vi "reward_behavior_0_6s_post_stim.vi"() -> ()   [LabVIEW 2019]
doc: "The myRIO Project template acquires acceleration data from the onboard accelerometer and displays the changes of acceleration values in a waveform chart."
uses:
  <vilib>/Analysis/Matrix/Datatypes/RealMatrix.ctl
  <vilib>/myRIO/Common/Instrument Driver Framework/myRIO v1.0/Encoder/typedefs/Encoder Signal Mode.ctl
  <vilib>/myRIO/Instrument Drivers/Onboard IO/Encoder/typedefs/Encoder Reference.ctl
  <vilib>/myRIO/Common/Instrument Driver Framework/Utilities/typedefs/myRIO Generic Hardware Reference.ctl
  <vilib>/myRIO/Common/Instrument Driver Framework/Utilities/typedefs/Hardware Version Enum.ctl
  <vilib>/myRIO/Common/Instrument Driver Framework/Utilities/typedefs/myRIO v1.0 Reference.ctl
  <vilib>/myRIO/Common/Instrument Driver Framework/Utilities/typedefs/Generic FPGA Reference.ctl
  <vilib>/myRIO/Common/Instrument Driver Framework/myRIO v1.0/Encoder/typedefs/Encoder Channels Enum.ctl
  <vilib>/myRIO/Common/Instrument Driver Framework/myRIO v1.0/Encoder/typedefs/Encoder Configuration v1.0.ctl
  <vilib>/userdefined/High Color/nirio_resource_hc.ctl
  <vilib>/myRIO/Instrument Drivers/Onboard IO/DIO/typedefs/DIO Reference.ctl
  <vilib>/myRIO/Common/Instrument Driver Framework/myRIO v1.0/DIO/typedefs/DIO Channels List.ctl
  <vilib>/myRIO/Common/Instrument Driver Framework/myRIO v1.0/DIO/typedefs/DIO Channels Enum.ctl
  <vilib>/myRIO/Common/Instrument Driver Framework/Utilities/vis/Is FPGA Ref Available.vi
  <vilib>/myRIO/Common/Instrument Driver Framework/myRIO v1.0/Encoder/vis/myRIO v1.1 Open Encoder.vi
  <vilib>/myRIO/Instrument Drivers/Onboard IO/Encoder/vis/Read.vi
  <vilib>/myRIO/Common/Instrument Driver Framework/myRIO v1.0/DIO/vis/myRIO v1.1 Open DIO.vi
  <vilib>/myRIO/Instrument Drivers/Onboard IO/DIO/vis/Write.vi
  <vilib>/myRIO/Instrument Drivers/Onboard IO/DIO/vis/Read.vi
  <vilib>/myRIO/Common/Instrument Driver Framework/Utilities/vis/Validate Channels.vi
  <vilib>/myRIO/Common/Instrument Driver Framework/myRIO v1.0/Encoder/vis/myRIO v1.0 Reserve Encoder.vi
  <vilib>/myRIO/Common/Instrument Driver Framework/myRIO v1.0/DIO/vis/myRIO v1.0 Reserve DIO.vi
  <vilib>/myRIO/Common/Instrument Driver Framework/myRIO v1.0/Encoder/vis/myRIO v1.0 Build MUX Configuration Encoder.vi
  <vilib>/myRIO/Common/Instrument Driver Framework/myRIO v1.0/Resource Manager/vis/myRIO v1.0 Reserve Channel List.vi
  <vilib>/myRIO/Common/Instrument Driver Framework/myRIO v1.0/DIO/vis/myRIO v1.0 Build MUX Configuration DIO.vi
  <vilib>/myRIO/Common/Instrument Driver Framework/myRIO v1.0/Resource Manager/vis/myRIO v1.0 Create Configuration List.vi
  <vilib>/myRIO/Common/Instrument Driver Framework/myRIO v1.0/Resource Manager/vis/myRIO v1.0 Reserve Channel.vi
  <vilib>/myRIO/Common/Instrument Driver Framework/myRIO v1.0/Resource Manager/vis/myRIO v1.0 Unreserve Channel.vi
  <vilib>/myRIO/Common/Instrument Driver Framework/myRIO v1.0/Resource Manager/vis/myRIO v1.0 Build Mutex Name.vi
  <vilib>/Utility/VariantDataType/GetNumericInfo.vi
  <vilib>/Utility/error.llb/Error Cluster From Error Code.vi
  <vilib>/myRIO/Common/Instrument Driver Framework/myRIO v1.0/myRIO v1.1 Open.vi
  <vilib>/myRIO/Common/Instrument Driver Framework/Utilities/vis/IO Manager.vi
  <vilib>/myRIO/Common/Instrument Driver Framework/Utilities/vis/Configuration Manager.vi
  <vilib>/myRIO/Common/Instrument Driver Framework/myRIO v1.0/Resource Manager/vis/myRIO v1.0 Configure IO.vi
  <vilib>/myRIO/Common/Instrument Driver Framework/myRIO v1.0/myRIO v1.0 Close.vi
  <vilib>/myRIO/Common/Instrument Driver Framework/myRIO v1.0/Encoder/vis/myRIO v1.0 Configure Encoder.vi
  <vilib>/myRIO/Common/Instrument Driver Framework/myRIO v1.0/Encoder/vis/myRIO v1.0 Read Encoder.vi
  <vilib>/myRIO/Common/Instrument Driver Framework/myRIO v1.0/DIO/vis/myRIO v1.0 Read DIO.vi
  <vilib>/myRIO/Common/Instrument Driver Framework/myRIO v1.0/DIO/vis/myRIO v1.0 Write DIO.vi
  <vilib>/myRIO/Express VI/Onboard IO/Encoder/Encoder Express VI.xnode
  <vilib>/myRIO/Instrument Drivers/Onboard IO/Encoder/vis/myRIO Encoder Open.xnode
  <vilib>/myRIO/Express VI/Onboard IO/DI/DI Express VI.xnode
  <vilib>/myRIO/Instrument Drivers/Onboard IO/DIO/vis/myRIO DIO Open.xnode
  <vilib>/myRIO/Express VI/Onboard IO/DO/DO Express VI.xnode
  <vilib>/myRIO/Instrument Drivers/Onboard IO/Encoder/Encoder.lvlib
  <vilib>/myRIO/Instrument Drivers/Onboard IO/DIO/DIO.lvlib
  <vilib>/Analysis/Matrix/NI_Matrix.lvlib
panel:
  out "Rewarded trials":dbl[](array[numeric])
  out "Rewards":u16
  out "Active Trial":bool
  out "Array temp2":T1
  out "Stimuli Loaded":bool
  out "Stim_ID":dbl[](array[numeric])
  out "Reward_mat":dbl[](array[numeric])
  out "Reward":bool=TRUE
  out "Frame clock":i32
  out "Licks":u32
  out "Lick":bool
  out "Time":dbl
  out "Stop":bool
  in  "Frames to collect":u32
  out "Overflow?":bool
  out "Counter Value":i32
  out "Velocity":dbl
  out "Velocity Plot":dbl[](graph)
  out "Velocity array":dbl[](array[numeric])
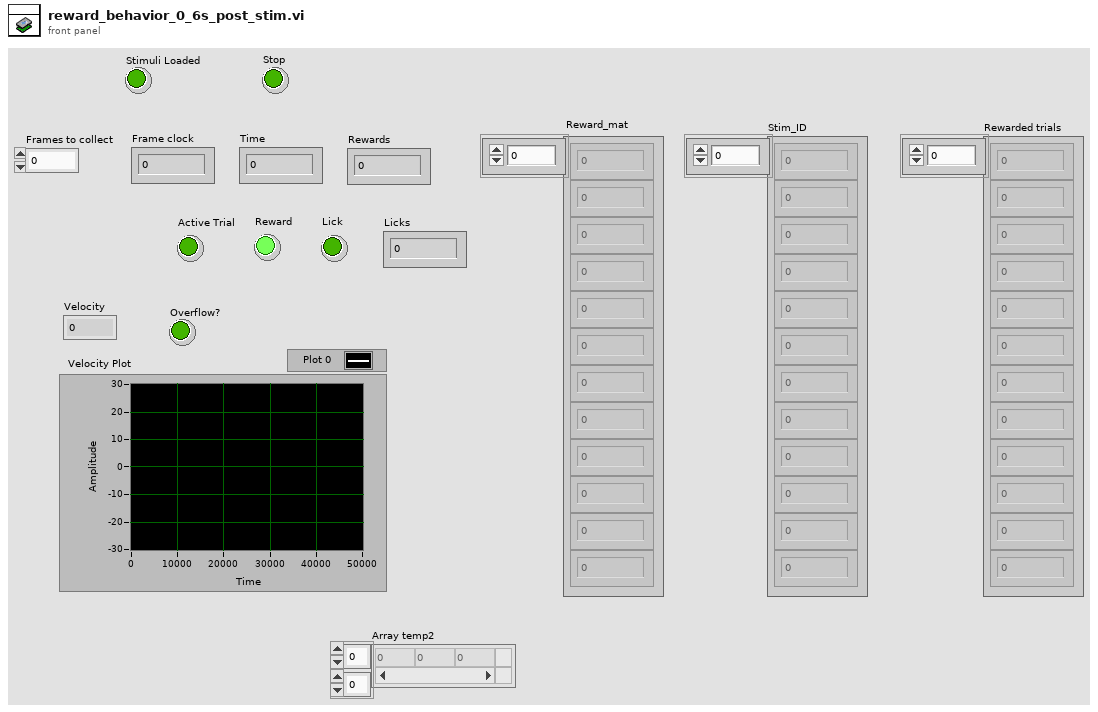
[diagram p1: front panel]
types:
  T1 = typedef "NI_Matrix.lvlib/RealMatrix.ctl" = dbl[][]
  T2 = typedef "Encoder.lvlib/Encoder Reference.ctl" = cluster{"myRIO Reference":T3, "Encoder Channels Enum":T7}
  T3 = typedef "myRIO Generic Hardware Reference.ctl" = cluster{"myRIO Model":T4, "myRIO Hardware Reference":T5}
  T4 = typedef "Hardware Version Enum.ctl" = enum16{"Unknown", "myRIO-1900", "myRIO-1950", "roboRIO", "NI ELVIS RIO CM", "ELVIS III"}
  T5 = typedef "myRIO v1.0 Reference.ctl" = cluster{"Generic FPGA Reference":T6, "Allow multiple opens":bool}
  T6 = typedef "Generic FPGA Reference.ctl" = refnum<k20>
  T7 = typedef "Encoder Channels Enum.ctl" = enum16{"Not Connected", "C/ENC0", "C/ENC1", "A/ENC", "A/ENC0", "A/ENC1", "A/ENC2", "A/ENC3", "A/ENC4", "A/ENC5", "A/ENC6", "A/ENC7", "A/ENC8", "A/ENC9", "B/ENC", "B/ENC0", "B/ENC1", "B/ENC2", "B/ENC3", "B/ENC4", "B/ENC5", "B/ENC6", "B/ENC7", "B/ENC8", "B/ENC9", "DIO/ENC0", "DIO/ENC1", "DIO/ENC2", "DIO/ENC3", "DIO/ENC4"}
  T8 = typedef "Encoder Signal Mode.ctl" = enum16{"Quadrature phase signal", "Step and direction signal"}
  T9 = typedef "nirio_resource_hc.ctl" = tag
  T10 = typedef "DIO.lvlib/DIO Reference.ctl" = cluster{"myRIO Reference":T3, "DIO Channels List":T11}
  T11 = typedef "DIO Channels List.ctl" = T12[]
  T12 = typedef "DIO Channels Enum.ctl" = enum16{"Not Connected", "C/DIO0", "C/DIO1", "C/DIO2", "C/DIO3", "C/DIO4", "C/DIO5", "C/DIO6", "C/DIO7", "A/DIO0", "A/DIO1", "A/DIO2", "A/DIO3", "A/DIO4", "A/DIO5", "A/DIO6", "A/DIO7", "A/DIO8", "A/DIO9", "A/DIO10", "A/DIO11", "A/DIO12", "A/DIO13", "A/DIO14", "A/DIO15", "A/DIO16", "A/DIO17", "A/DIO18", "A/DIO19", "B/DIO0", "B/DIO1", "B/DIO2", "B/DIO3", "B/DIO4", "B/DIO5", "B/DIO6", "B/DIO7", "B/DIO8", "B/DIO9", "B/DIO10", "B/DIO11", "B/DIO12", "B/DIO13", "B/DIO14", "B/DIO15", "B/DIO16", "B/DIO17", "B/DIO18", "B/DIO19", "LED0", "LED1", "LED2", "LED3", "Button0", "DIO/DIO0", "DIO/DIO1", "DIO/DIO2", "DIO/DIO3", "DIO/DIO4", "DIO/DIO5", "DIO/DIO6", "DIO/DIO7", "DIO/DIO8", "DIO/DIO9", "SPI/CS0", "SPI/CS1", "SPI/CS2", "SPI/CS3", "LED RADIO (Green)", "LED RADIO (Red)", "LED COMM (Green)", "LED COMM (Red)", "LED MODE (Green)", "LED MODE (Red)"}
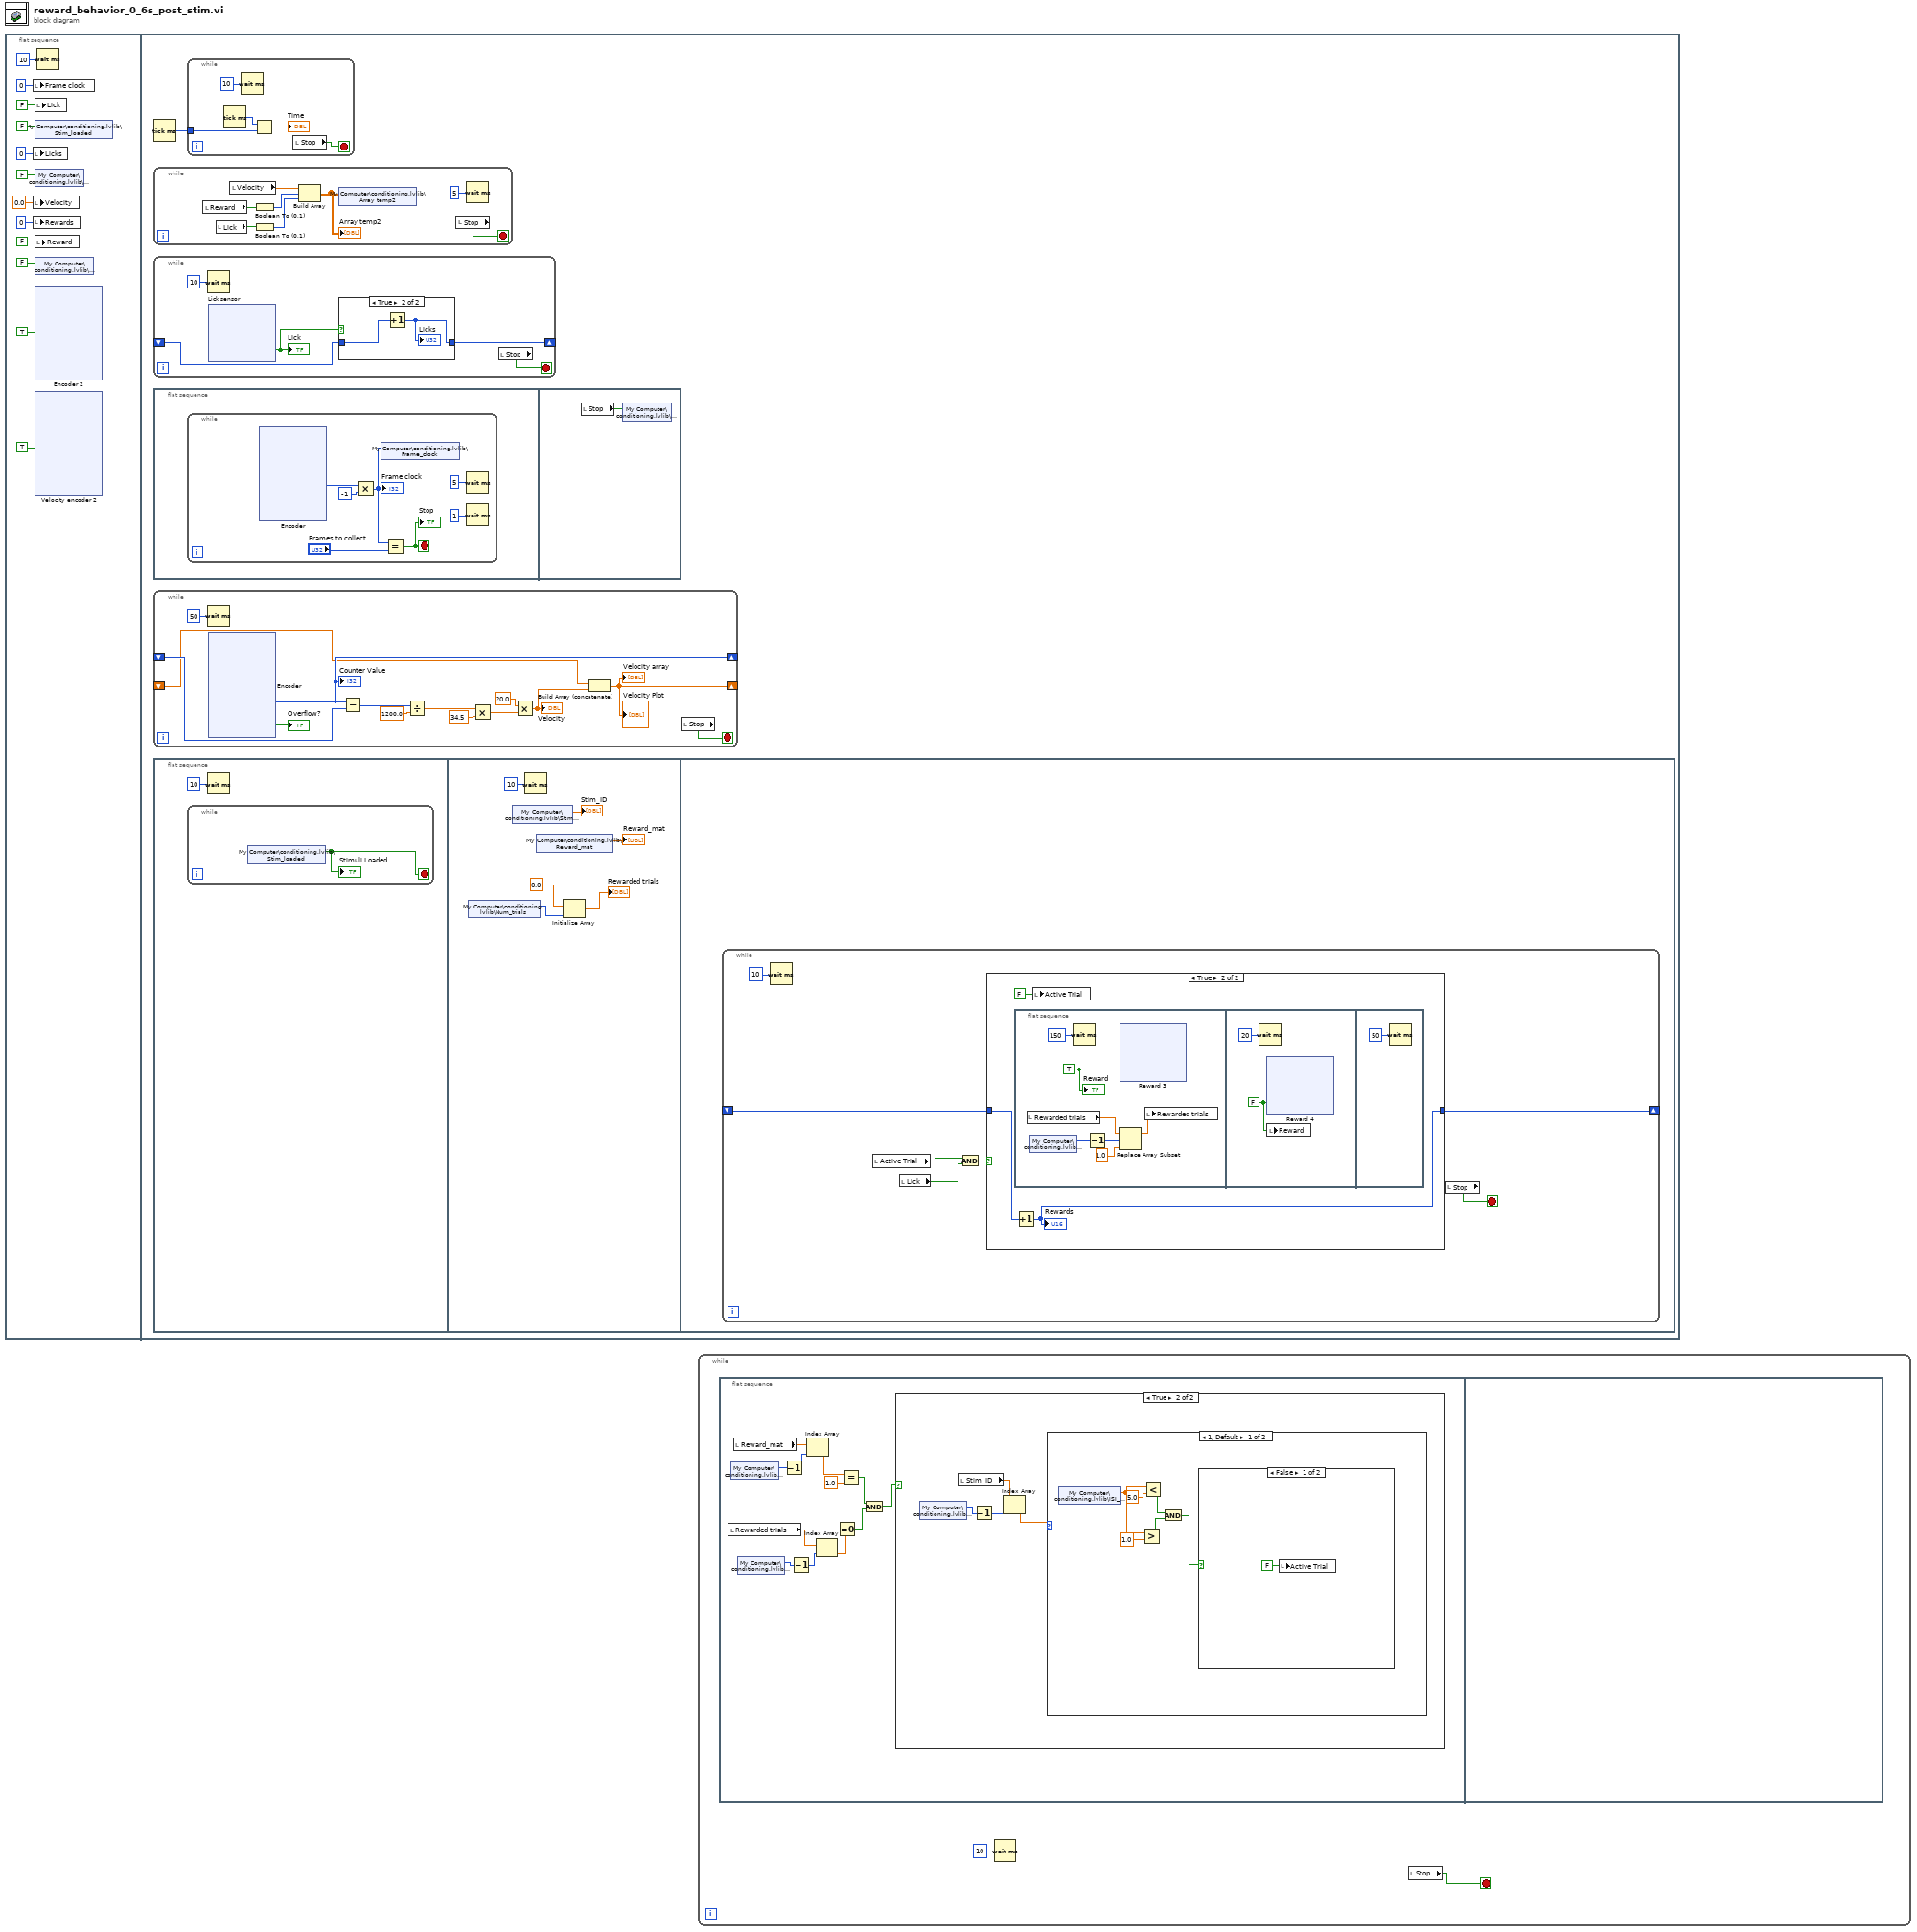
[diagram p0: block diagram]
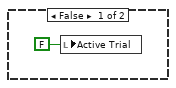
[diagram p2: hidden frame]
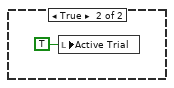
[diagram p3: hidden frame]
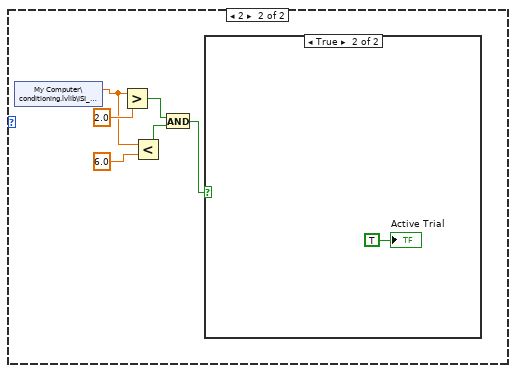
[diagram p4: hidden frame]
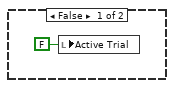
[diagram p5: hidden frame]
diagram:
  n1 = flat-sequence {
    frame #0 {
      n2 = local write "Frame clock"(u32 0 ("Frames")) -> ()
      n3 = local write "Licks"(u32 0 ("Licks")) -> ()
      n4 = local write "Velocity"(0.0 ("Velocity")) -> ()
      n5 = local write "Rewards"(u16 0 ("Rewards")) -> ()
      n6 = local write "Lick"(FALSE ("Lick")) -> ()
      n7 = shared-variable "My Computer\\conditioning.lvlib\\Stim_loaded"(FALSE ("Stim_loaded")) -> ()  [unwired: 1 in, 1 out]
      n8 = shared-variable "My Computer\\conditioning.lvlib\\Stop"(FALSE ("Stop")) -> ()  [unwired: 1 in, 1 out]
      n9 = local write "Reward"(FALSE ("Give reward")) -> ()
      n10 = shared-variable "My Computer\\conditioning.lvlib\\Display"(FALSE ("Display")) -> ()  [unwired: 1 in, 1 out]
      n11 = xnode "Encoder 2"("Reset Counter"=TRUE) -> ()  [unwired: 1 in, 4 out]
      n12 = xnode "Velocity encoder 2"("Reset Counter"=TRUE) -> ()  [unwired: 1 in, 4 out]
      n13 = Wait (ms)(milliseconds to wait=u32 10) -> ()  [unwired: 1 out]
    }
    frame #1 {
      n14 = Tick Count (ms)() -> (millisecond timer value=w105:u32)
      n15 = while {
        stop <- w107 stop-if-true
        n16 = local read "Reward"() -> (w112:bool)
        n17 = local read "Lick"() -> (w113:bool)
        n18 = local read "Velocity"() -> (w111:dbl)
        n19 = Boolean To (0,1)(Boolean=w112) -> (0, 1=w110:i16)
        n20 = Boolean To (0,1)(Boolean=w113) -> (0, 1=w109:i16)
        n21 = Build Array(w111, w110, w109) -> (w106:T1)
        "Array temp2" <- w106
        n22 = shared-variable "My Computer\\conditioning.lvlib\\Array temp2"(w106) -> ()  [unwired: 1 in, 1 out]
        n23 = local read "Stop"() -> (w107:bool)
        n24 = Wait (ms)(milliseconds to wait=u32 5) -> ()  [unwired: 1 out]
      }
      n25 = while {
        shift-right: [w269] -> _
        shift-left: _ -> [w268]
        stop <- w267 stop-if-true
        n26 = Wait (ms)(milliseconds to wait=u32 10) -> ()  [unwired: 1 out]
        n27 = xnode "Lick sensor"() -> ("C/DIO1 (DIO1)"=w270:bool)  [unwired: 1 in, 1 out]
        "Lick" <- w270
        n28 = case shown="True" w270 {
          tunnel: [w272 w274] -> w269
          tunnel: w268 -> [w272 w273]
          frame False {
          }
          frame True {
            n29 = Increment(x=w273) -> (x+1=w274:u32)
            "Licks" <- w274
          }
        }
        n30 = local read "Stop"() -> (w267:bool)
      }
      n31 = flat-sequence {
        frame #0 {
          n32 = while {
            stop <- w214 stop-if-true
            n33 = xnode "Encoder"() -> ("Counter Value"=w218:i32)  [unwired: 2 in, 3 out]
            n34 = Multiply(x=w218, y=-1) -> (x*y=w213:i32)
            "Frame clock" <- w213
            n35 = shared-variable "My Computer\\conditioning.lvlib\\Frame_clock"(w213) -> ()  [unwired: 1 in, 1 out]
            n36 = Equal?(x=w213, y="Frames to collect") -> (x = y?=w214:bool)
            "Stop" <- w214
            n37 = Wait (ms)(milliseconds to wait=u32 5) -> ()  [unwired: 1 out]
            n38 = Wait (ms)(milliseconds to wait=u32 1) -> ()  [unwired: 1 out]
          }
        }
        frame #1 {
          n39 = local read "Stop"() -> (w266:bool)
          n40 = shared-variable "My Computer\\conditioning.lvlib\\Stop"(w266) -> ()  [unwired: 1 in, 1 out]
        }
      }
      n41 = while {
        shift-right: [w320] -> _
        shift-left: _ -> [w321]
        shift-right: [w312] -> _
        shift-left: _ -> [w311]
        stop <- w310 stop-if-true
        n42 = Wait (ms)(milliseconds to wait=u32 50) -> ()  [unwired: 1 out]
        n43 = xnode "Encoder"() -> ("Counter Value"=w320:i32, "Overflow?"=→"Overflow?":bool)  [unwired: 2 in, 2 out]
        "Counter Value" <- w320
        n44 = Subtract(x=w320, y=w321) -> (x-y=w313:i32)
        n45 = Divide(x=w313, y=1200.0 ("600")) -> (x/y=w318:dbl)
        n46 = Multiply(x=w318, y=34.5) -> (x*y=w316:dbl)
        n47 = Multiply(x=20.0, y=w316) -> (x*y=w314:dbl)
        "Velocity" <- w314
        n48 = Build Array (concatenate)(w311, w314) -> (w312:dbl[])
        "Velocity Plot" <- w312
        "Velocity array" <- w312
        n49 = local read "Stop"() -> (w310:bool)
      }
      n50 = flat-sequence {
        frame #0 {
          n51 = while {
            stop <- w115 stop-if-true
            n52 = shared-variable "My Computer\\conditioning.lvlib\\Stim_loaded"() -> (w115:bool)  [unwired: 1 in, 1 out]
            "Stimuli Loaded" <- w115
          }
          n53 = Wait (ms)(milliseconds to wait=u32 10) -> ()  [unwired: 1 out]
        }
        frame #1 {
          n54 = shared-variable "My Computer\\conditioning.lvlib\\Num_trials"() -> (w118:u32)  [unwired: 1 in, 1 out]
          n55 = shared-variable "My Computer\\conditioning.lvlib\\Stim_ID"() -> (→"Stim_ID":dbl[])  [unwired: 1 in, 1 out]
          n56 = Wait (ms)(milliseconds to wait=u32 10) -> ()  [unwired: 1 out]
          n57 = shared-variable "My Computer\\conditioning.lvlib\\Reward_mat"() -> (→"Reward_mat":dbl[])  [unwired: 1 in, 1 out]
          n58 = Initialize Array(0.0 ("element"), w118) -> (→"Rewarded trials":dbl[])
        }
        frame #2 {
          n59 = while {
            shift-right: [w125] -> _
            shift-left: _ -> [w124]
            stop <- w128 stop-if-true
            n60 = Wait (ms)(milliseconds to wait=u32 10) -> ()  [unwired: 1 out]
            n61 = local read "Active Trial"() -> (w122:bool)
            n62 = local read "Lick"() -> (w123:bool)
            n63 = And(x=w122, y=w123) -> (x .and. y?=w126:bool)
            n64 = case shown="True" w126 {
              tunnel: [w129 w132] -> w125
              tunnel: w124 -> [w129 w131]
              frame False {
              }
              frame True {
                n65 = flat-sequence {
                  frame #0 {
                    w138 = TRUE ("C/DIO0 (DIO0)")
                    n66 = local read "Rewarded trials"() -> (w135:dbl[])
                    n67 = shared-variable "My Computer\\conditioning.lvlib\\Trial"() -> (w137:u32)  [unwired: 1 in, 1 out]
                    n68 = Wait (ms)(milliseconds to wait=u32 150) -> ()  [unwired: 1 out]
                    n69 = Decrement(x=w137) -> (x-1=w136:u32)
                    n70 = Replace Array Subset(array=w135, new element=1.0 ("new element/subarray"), index=w136) -> (w133:dbl[])
                    n71 = xnode "Reward 3"("C/DIO0 (DIO0)"=w138) -> ()  [unwired: 1 in, 1 out]
                    n72 = local write "Rewarded trials"(w133) -> ()
                    "Reward" <- w138
                  }
                  frame #1 {
                    w176 = FALSE ("C/DIO0 (DIO0)")
                    n73 = Wait (ms)(milliseconds to wait=u32 20) -> ()  [unwired: 1 out]
                    n74 = xnode "Reward 4"("C/DIO0 (DIO0)"=w176) -> ()  [unwired: 1 in, 1 out]
                    n75 = local write "Reward"(w176) -> ()
                  }
                  frame #2 {
                    n76 = Wait (ms)(milliseconds to wait=u32 50) -> ()  [unwired: 1 out]
                  }
                }
                n77 = Increment(x=w131) -> (x+1=w132:u16)
                "Rewards" <- w132
                n78 = local write "Active Trial"(FALSE ("Active Trial")) -> ()
              }
            }
            n79 = local read "Stop"() -> (w128:bool)
          }
        }
      }
      n80 = while {
        tunnel: w105 -> [w373]
        stop <- w370 stop-if-true
        n81 = Tick Count (ms)() -> (millisecond timer value=w374:u32)
        n82 = Wait (ms)(milliseconds to wait=u32 10) -> ()  [unwired: 1 out]
        n83 = Subtract(x=w374, y=w373) -> (x-y=→"Time":u32)
        n84 = local read "Stop"() -> (w370:bool)
      }
    }
  }
  n85 = while {
    stop <- w376 stop-if-true
    n86 = flat-sequence {
      frame #0 {
        n87 = local read "Rewarded trials"() -> (w383:dbl[])
        n88 = shared-variable "My Computer\\conditioning.lvlib\\Trial"() -> (w386:u32)  [unwired: 1 in, 1 out]
        n89 = local read "Reward_mat"() -> (w385:dbl[])
        n90 = shared-variable "My Computer\\conditioning.lvlib\\Trial"() -> (w382:u32)  [unwired: 1 in, 1 out]
        n91 = Decrement(x=w386) -> (x-1=w387:u32)
        n92 = Decrement(x=w382) -> (x-1=w381:u32)
        n93 = Index Array(array=w385, index=w387) -> (element=w388:dbl)
        n94 = Index Array(array=w383, index=w381) -> (element=w380:dbl)
        n95 = Equal To 0?(x=w380) -> (x = 0?=w379:bool)
        n96 = Equal?(x=w388, y=1.0) -> (x = y?=w378:bool)
        n97 = And(x=w378, y=w379) -> (x .and. y?=w377:bool)
        n98 = case shown="True" w377 {
          frame False {
            n99 = local write "Active Trial"(FALSE ("Active_trial")) -> ()
          }
          frame True {
            n100 = shared-variable "My Computer\\conditioning.lvlib\\Trial"() -> (w391:u32)  [unwired: 1 in, 1 out]
            n101 = local read "Stim_ID"() -> (w393:dbl[])
            n102 = Decrement(x=w391) -> (x-1=w392:u32)
            n103 = Index Array(array=w393, index=w392) -> (element=w390:dbl)
            n104 = case shown="1, Default" w390 {
              frame 1, Default {
                n105 = shared-variable "My Computer\\conditioning.lvlib\\ISI_Time"() -> (w398:dbl)  [unwired: 1 in, 1 out]
                n106 = Greater?(x=w398, y=1.0) -> (0:w395:bool)
                n107 = Less?(x=w398, y=5.0) -> (x < y?=w396:bool)
                n108 = And(x=w396, y=w395) -> (x .and. y?=w394:bool)
                n109 = case shown="False" w394 {
                  frame False {
                    n110 = local write "Active Trial"(FALSE ("Active Trial")) -> ()
                  }
                  frame True {
                    n111 = local write "Active Trial"(TRUE ("Active Trial")) -> ()
                  }
                }
              }
              frame 2 {
                n112 = shared-variable "My Computer\\conditioning.lvlib\\ISI_Time"() -> (w406:dbl)  [unwired: 1 in, 1 out]
                n113 = Greater?(x=w406, y=2.0) -> (0:w404:bool)
                n114 = Less?(x=w406, y=6.0) -> (x < y?=w403:bool)
                n115 = And(x=w404, y=w403) -> (x .and. y?=w402:bool)
                n116 = case shown="True" w402 {
                  frame False {
                    n117 = local write "Active Trial"(FALSE ("Active Trial")) -> ()
                  }
                  frame True {
                    "Active Trial" <- TRUE ("Active Trial")
                  }
                }
              }
            }
          }
        }
      }
      frame #1 {
      }
    }
    n118 = Wait (ms)(milliseconds to wait=u32 10) -> ()  [unwired: 1 out]
    n119 = local read "Stop"() -> (w376:bool)
  }
